vi "Icon_Extract Icon.vi"(0 "VI REF":refnum<vi>, 3 "Error":errorcluster, 4 "Path":path) -> (7 "VI REF Out":refnum<vi>, 9 "ImageData Out":T1, 10 "Error Out":errorcluster)   [LabVIEW 2009]
doc: "Extracts Image data from a Vi reference"
uses:
  Controls/Cluster/Cluster_Image Data.ctl
  Controls/Cluster/CLuster_Selectoin Box.ctl
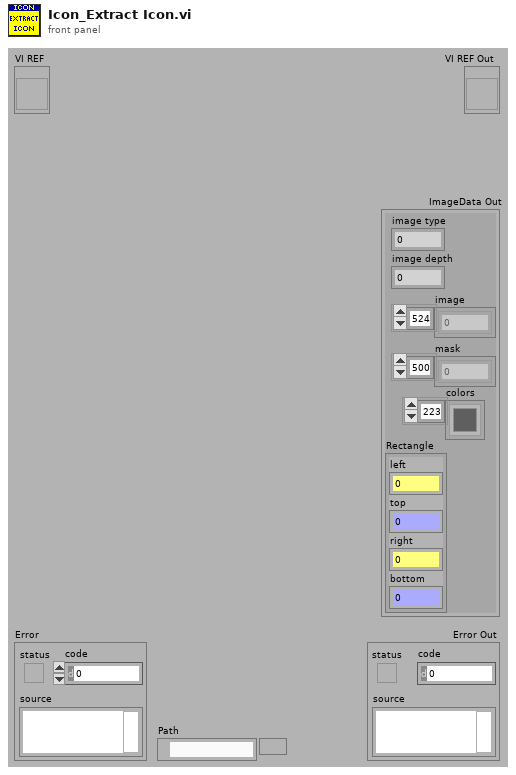
[diagram p1: front panel]
types:
  T1 = typedef "Cluster_Image Data.ctl" = cluster{"image type":i32, "image depth":i32, "image":u8[], "mask":u8[], "colors":u32[], "Rectangle":T2}
  T2 = typedef "CLuster_Selectoin Box.ctl" = cluster{"left":i16, "top":i16, "right":i16, "bottom":i16}
  T3 = typedef "imagedata.ctl" = cluster{"image type":i32, "image depth":i32, "image":u8[], "mask":u8[], "colors":u32[], "Rectangle":cluster{"left":i16, "top":i16, "right":i16, "bottom":i16}}
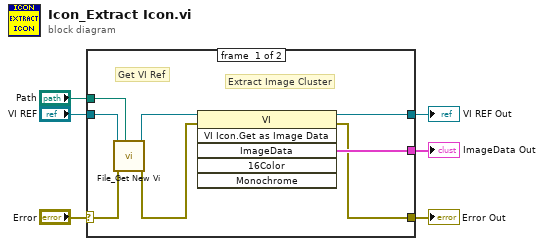
[diagram p0: block diagram]
diagram:
  n1 = case shown="No Error" "Error" {
    selector: "Error" -> [w7 w15]
    tunnel: "Path" -> [w14 _]
    tunnel: "VI REF" -> [w13 w16]
    tunnel: [w11 _] -> w4
    tunnel: [w10 w16] -> w3
    tunnel: [w9 w15] -> w2
    frame #0 {
      # "Extract Image Cluster"
      # "Get VI Ref"
      n2 = call "File_Get New Vi.vi"("VI REF"=w13, "Error"=w7, "Path"=w14) -> ("VI REF Out"=w8:refnum<vi>, "Error Out"=w12:errorcluster)  [unwired: 5 in, 1 out]
      n3 = invoke class="VI" method="VI Icon.Get as Image Data"(reference=w8, error in=w12) -> (reference out=w10:refnum<vi>, error out=w9:errorcluster, "ImageData"=w11:T3)  [unwired: 4 in, 3 out]
    }
    frame #1 {
    }
  }
  "ImageData Out" <- w4
  "VI REF Out" <- w3
  "Error Out" <- w2
